vi "Resolution Check Popup.vi"(8 "error in":errorcluster, 10 "VI in":refnum<vi>, 11 "SR for Check":T1 {"Creation Date" format="%<%x>T"; "Last Updated" format="%<%x>T"}) -> (0 "error out":errorcluster, 2 "Passed Off?":bool, 3 "Window Closed?":bool)   [LabVIEW 2018]
uses:
  Type Defs/SR Cluster.ctl
  Type Defs/SR Status.ctl
  <vilib>/Utility/miscctls.llb/LVPointTypeDef.ctl
panel:
  in  "Resolved":bool
  in  "Passed Off":bool
  out "SR Information":string
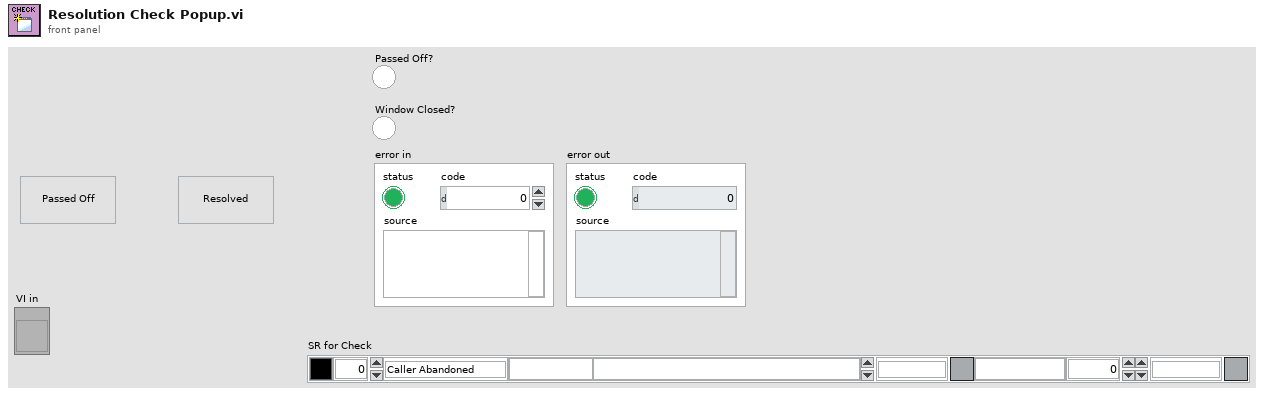
[diagram p1: front panel]
types:
  T1 = typedef "SR Cluster.ctl" = cluster{"Color":u32, "SR Number":i32, "SR Status":T2, "SR Type":string, "Summary":string, "Last Updated":timestamp, "Service Level":string, "Days Open":dbl, "Creation Date":timestamp}
  T2 = typedef "SR Status.ctl" = enum16{"Caller Abandoned", "Created in Error", "Expired", "Forum Resolved AE", "Forum Resolved Customer", "IN WORK", "IN WORK Collab with AES", "IN WORK Collab with PSE", "IN WORK Collab with SE", "IN WORK Customer Added Note", "IN WORK Escalation", "IN WORK Wait on Customer", "Open", "Potentially Resolved", "Presumed Resolved", "RMA Approved for Return", "Resolved", "Passed Off"}
  T3 = typedef "LVPointTypeDef.ctl" = cluster{"Horizontal":i16, "Vertical":i16}
  T4 = typedef "LVRectTypeDef.ctl" = cluster{"Left":i16, "Top":i16, "Right":i16, "Bottom":i16}
  T5 = typedef "LVBoundsTypeDef.ctl" = cluster{"Width":u32, "Height":u32}
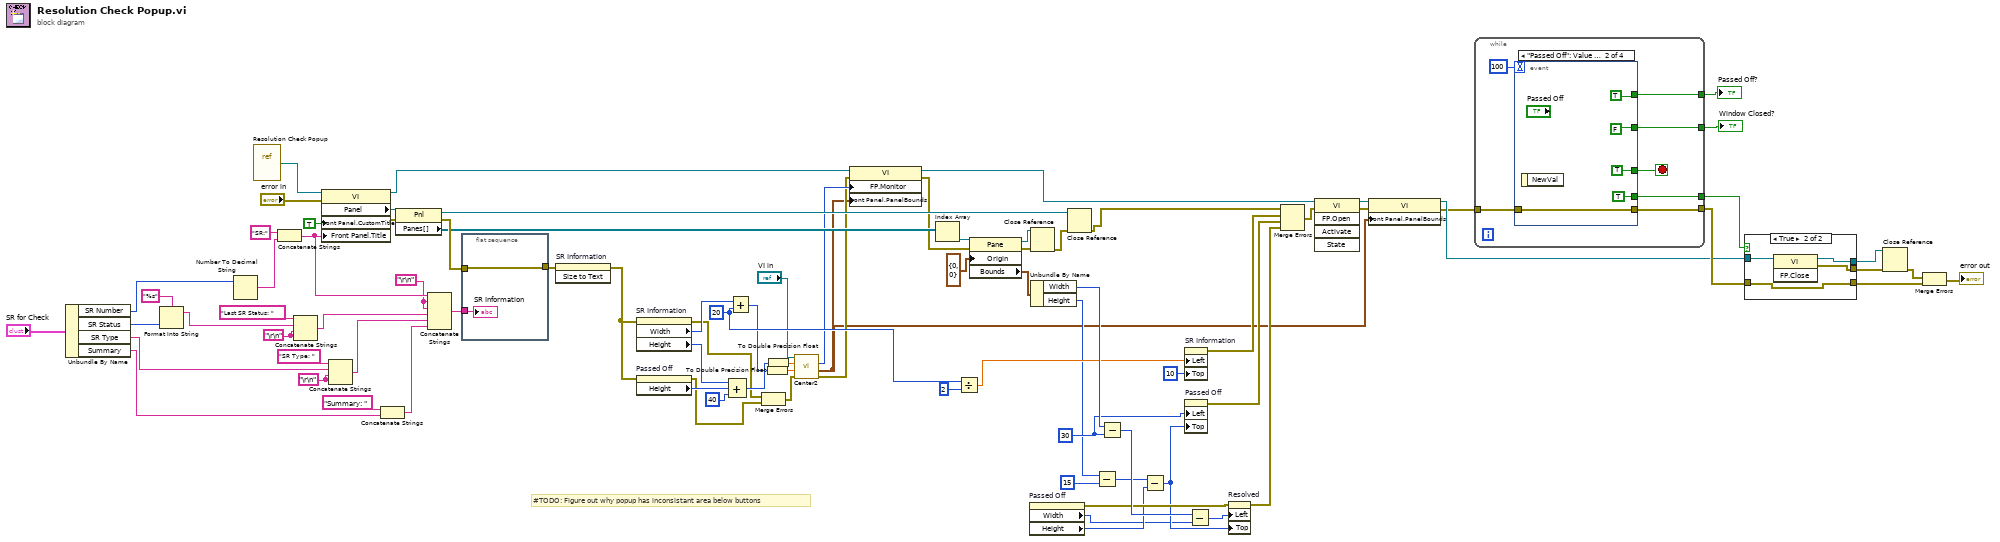
[diagram p0: block diagram]
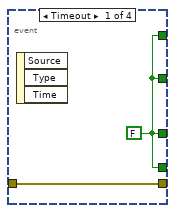
[diagram p3: hidden frame]
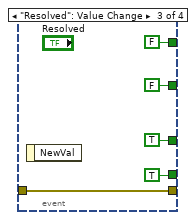
[diagram p4: hidden frame]
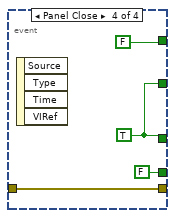
[diagram p5: hidden frame]
diagram:
  w50 = 30 ("Position:Left")
  w49 = u32 20 ("y")
  w46 = "\r\n"
  w45 = "\r\n"
  w42 = "\r\n"
  # "#TODO: Figure out why popup has inconsistant area below buttons"
  n1 = Unbundle By Name("SR for Check") -> ("SR Number"=w67:i32, "SR Status"=w26:T2, "SR Type"=w60:string, "Summary"=w61:string)
  n2 = Format Into String(format string="%s", w26) -> (resulting string=w24:string)  [unwired: 2 in, 1 out]
  n3 = Number To Decimal String(number=w67) -> (decimal integer string=w71:string)  [unwired: 1 in]
  n4 = vi-ref "Resolution Check Popup.vi"() -> (w79:refnum<vi>)
  n5 = Concatenate Strings("SR:" ("string"), w71) -> (w66:string)
  n6 = Concatenate Strings("Last SR Status: " ("string"), w24, w45, w45) -> (w44:string)
  n7 = property class="VI"(reference=w79, error in="error in", "Front Panel.CustomTitle"=TRUE ("Front Panel Window:Custom Title"), "Front Panel.Title"=w66) -> (reference out=w59:refnum<vi>, error out=w80:errorcluster, "Panel"=w81:refnum<vi>)
  n8 = Concatenate Strings("SR Type: " ("string"), w60, w46, w46) -> (w43:string)
  n9 = Concatenate Strings("Summary: " ("string"), w61) -> (w41:string)
  n10 = property class="Pnl"(reference=w81, error in=w80) -> (reference out=w82:refnum<vi>, error out=w70:errorcluster, "Panes[]"=w69:refnum<vi>[])
  n11 = Concatenate Strings(w66, w42, w42, w44, w43, w41) -> (w65:string)
  n12 = flat-sequence {
    tunnel: [w89] -> w28
    tunnel: w70 -> [w89]
    tunnel: w65 -> [w88]
    frame #0 {
      "SR Information" <- w88
    }
  }
  n13 = invoke on="SR Information" class="Str" method="Size to Text"(error in=w28) -> (error out=w23:errorcluster)  [unwired: 2 in, 2 out]
  n14 = property on="SR Information" class="Str"(error in=w23) -> (error out=w16:errorcluster, "Width"=w29:u32, "Height"=w30:u32)  [unwired: 1 in, 1 out]
  n15 = property on="Passed Off" class="Bool"(error in=w23) -> (error out=w17:errorcluster, "Height"=w57:u32)  [unwired: 1 in, 1 out]
  n16 = Add(x=w29, y=w49) -> (x+y=w19:u32)
  n17 = Compound Arithmetic op=ADD(w30, w57, u32 40 ("y")) -> (w20:u32)
  n18 = Merge Errors(w16, w17) -> (w15:errorcluster)
  n19 = To Double Precision Float(number=w19) -> (double precision float=w21:dbl)
  n20 = To Double Precision Float(number=w20) -> (double precision float=w22:dbl)
  n21 = call "Center2.vi"("error in (no error)"=w15, "Width"=w21, "Height"=w22, "VI in"="VI in") -> ("error out"=w14:errorcluster, "New Bounds"=w1:T4, "Active Monitor"=w18:u16)  [unwired: 5 in]
  n22 = property class="VI"(reference=w59, error in=w14, "FP.Monitor"=w18, "Front Panel.PanelBounds"=w1) -> (reference out=w11:refnum<vi>, error out=w58:errorcluster)
  n23 = Index Array(array=w69) -> (element=w87:refnum<vi>)  [unwired: 1 in]
  n24 = Divide(x=w49, y=u32 2) -> (x/y=w47:dbl)
  n25 = property class="Pane"(reference=w87, error in=w58, "Origin"=T3 {"Horizontal"=0, "Vertical"=0}) -> (reference out=w85:refnum<vi>, error out=w84:errorcluster, "Bounds"=w73:T5)
  n26 = property on="Passed Off" class="Bool"() -> (error out=w37:errorcluster, "Width"=w32:u32, "Height"=w33:u32)  [unwired: 2 in, 1 out]
  n27 = Close Reference(reference=w85, error in (no error)=w84) -> (error out=w83:errorcluster)
  n28 = Unbundle By Name(w73) -> ("Width"=w56:u32, "Height"=w36:u32)
  n29 = Close Reference(reference=w82, error in (no error)=w83) -> (error out=w12:errorcluster)
  n30 = Subtract(x=w36, y=u32 15) -> (x-y=w35:u32)
  n31 = Subtract(x=w56, y=w50) -> (x-y=w55:u32)
  n32 = Subtract(x=w35, y=w33) -> (x-y=w34:u32)
  n33 = property on="SR Information" class="Str"("Left"=w47, "Top"=10 ("Position:Top")) -> (error out=w53:errorcluster)  [unwired: 2 in, 1 out]
  n34 = property on="Passed Off" class="Bool"("Left"=w50, "Top"=w34) -> (error out=w52:errorcluster)  [unwired: 2 in, 1 out]
  n35 = Subtract(x=w55, y=w32) -> (x-y=w38:u32)
  n36 = property on="Resolved" class="Bool"(error in=w37, "Left"=w38, "Top"=w34) -> (error out=w51:errorcluster)  [unwired: 1 in, 1 out]
  n37 = Merge Errors(w12, w53, w52, w51) -> (w54:errorcluster)
  n38 = invoke class="VI" method="FP.Open"(reference=w11, error in=w54) -> (reference out=w5:refnum<vi>, error out=w2:errorcluster)  [unwired: 3 in, 3 out]
  n39 = property class="VI"(reference=w5, error in=w2, "Front Panel.PanelBounds"=w1) -> (reference out=w4:refnum<vi>, error out=w3:errorcluster)
  n40 = while {
    tunnel: w3 -> [w95]
    tunnel: [w96] -> w78
    tunnel: [w92] -> w75
    tunnel: [w91] -> w74
    tunnel: [w90] -> w6
    stop <- w93 stop-if-true
    n41 = event shown="[1] \"Passed Off\": Value Change" {
      selector: _ -> [_ _ _ _]
      dyn-events: _ -> [_ _ _ _]
      timeout: 100 -> [_ _ _ _]
      tunnel: [w98 w100 w105 w110] -> w96
      tunnel: w95 -> [w98 w100 w105 w110]
      tunnel: [w97 TRUE TRUE w112] -> w93
      tunnel: [w97 FALSE FALSE w112] -> w92
      tunnel: [w97 TRUE FALSE FALSE] -> w91
      tunnel: [w97 TRUE TRUE FALSE] -> w90
      event Timeout {
        w97 = FALSE
        n42 = event-data() -> ()  [unwired: 1 in, 3 out]
      }
      event "Passed Off": Value Change {
        n43 = event-data() -> ()  [unwired: 1 in, 1 out]
      }
      event "Resolved": Value Change {
        n44 = event-data() -> ()  [unwired: 1 in, 1 out]
      }
      event Panel Close {
        w112 = TRUE
        n45 = event-data() -> ()  [unwired: 1 in, 4 out]
      }
    }
  }
  "Passed Off?" <- w74
  "Window Closed?" <- w75
  n46 = case shown="True" w6 {
    tunnel: w78 -> [w113 w115]
    tunnel: w4 -> [w114 w118]
    tunnel: [w114 w117] -> w27
    tunnel: [w113 w116] -> w10
    tunnel: [w113 w115] -> w9
    frame False {
    }
    frame True {
      n47 = invoke class="VI" method="FP.Close"(reference=w118) -> (reference out=w117:refnum<vi>, error out=w116:errorcluster)  [unwired: 2 in, 1 out]
    }
  }
  n48 = Close Reference(reference=w27, error in (no error)=w10) -> (error out=w8:errorcluster)
  n49 = Merge Errors(w8, w9) -> (→"error out":errorcluster)
